vi "ScopeSignalManipulation_v1.vi"() -> ()   [LabVIEW 2018]
doc: "This example illustrates how to use autosetup and continuously acquires waveforms from a single channel using the following steps:\n\n1. Specify a valid VISA session. \n2. Specify a channel. \n3. Specify a time-out value for reading waveform.\n4. Run the VI. The graph displays the waveform you acquire."
uses:
  <vilib>/Analysis/baseanly.llb/Mean (DBL).vi
  <instrlib>/Tektronix DPO MSO 2000 4000 Series/Public/Data/Read (Single Waveform).vi
  <vilib>/Waveform/WDTFileIO.llb/Export Waveform To Spreadsheet File.vi
  <instrlib>/Tektronix DPO MSO 2000 4000 Series/Tektronix DPO MSO 2000 4000 Series.lvlib
  <vilib>/Analysis/NI_AALBase.lvlib
panel:
  in  "Tab Control":enum32{"Charge Amplifier", "Pulse Int"}(tab)=enum."Pulse Int"
  out "Charge Amp Signal (mV)":dbl=4.154735158126834 format="%#_6f"
  out "Number of Positrons":dbl=216046.22822259535
  out "Waveform Graph 2":waveform(dbl)(graph)={"t0"=timestamp(0 s since 1904-01-01), "dt"=4e-10, "Y"=array[5806 elements]}
  out "Base":dbl=-1.565120000000005e-08
  out "Signal":dbl=1.2079999999999996e-10
  out "Result (nVs)":dbl=15.77200000000005
  out "Mean BG":dbl=0.019374295870932312
  out "Mean ROI":dbl=0.015219560712805478
  out "BG ROI Length":i32=7314
  out "ROI Length":i32=2413
  out "I(BG Stop)":i32=495986
  out "I(BG start)":i32=488672
  out "I(stop)":i32=501340
  out "I(start)":i32=498927
  in  "Measurement Type":enum16{"Charge Amplifier", "Pulse Int"}(ring)=enum."Pulse Int"
  in  "Save waveform?":bool
  in  "acquire":bool=TRUE
  in  "milliseconds to wait":u32=100
  in  "Looping?":bool
  in  "stop":bool
  out "bkgd stop":dbl=0.000196584686774942
  out "bkgd start":dbl=0.00019546867749419954
  out "stop int":dbl=0.00020053596287703017
  out "start int":dbl=0.00019821345707656614
  in  "Channel (0: Channel 1)":u16(ring)=2 items=["Channel 1", "Channel 2", "Channel 3", "Channel 4", "Math", "Reference 1", "Reference 2", "Reference 3", "Reference 4"]
  in  "Maximum Time (10000ms)":u32=10000
  in  "VISA Resource Name":refnum<visa-resource-name>="mdo4034c"
  out "Waveform Graph":waveform(dbl)(graph)={"t0"=timestamp(-0.000197980000000042 s since 1904-01-01), "dt"=4e-10, "Y"=array[1000000 elements]}
  # "Region of Interest (ROI) Details"
  # "Time"
  # "Index"
  # "Length"
  # "Dashed cursors are the background, soild are the ROI"
  # "Use the solid ROI Cursors to define the region to integrate from the scope"
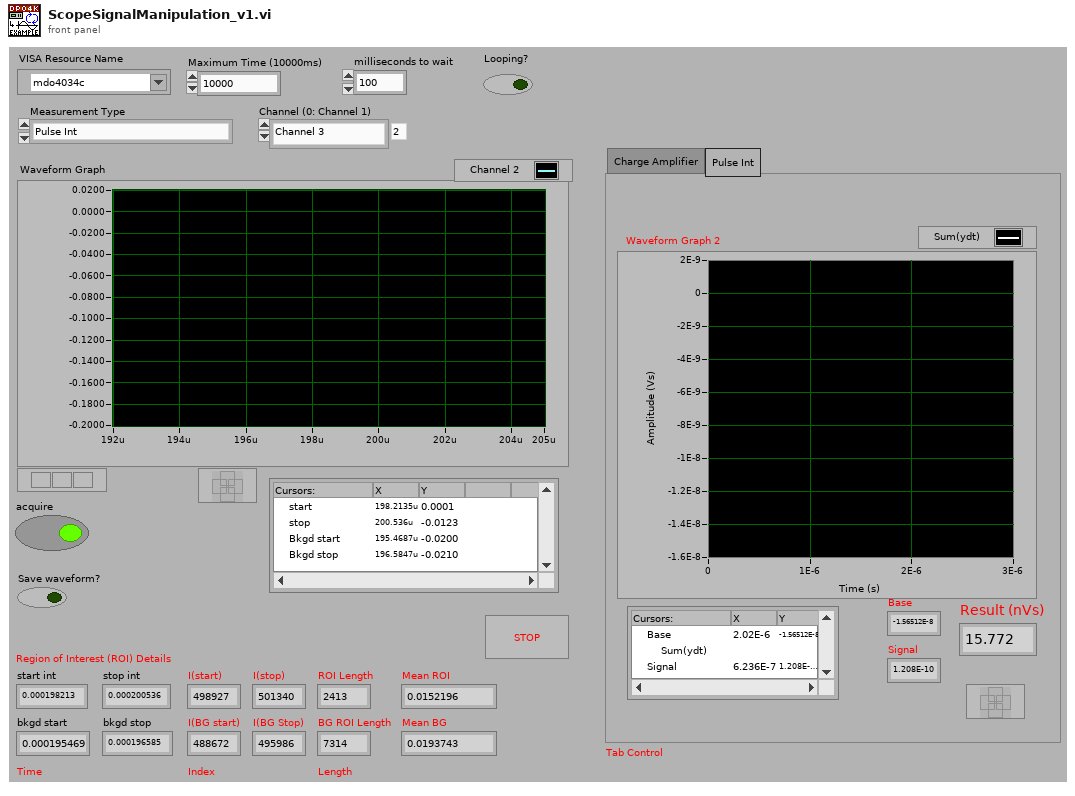
[diagram p1: front panel]
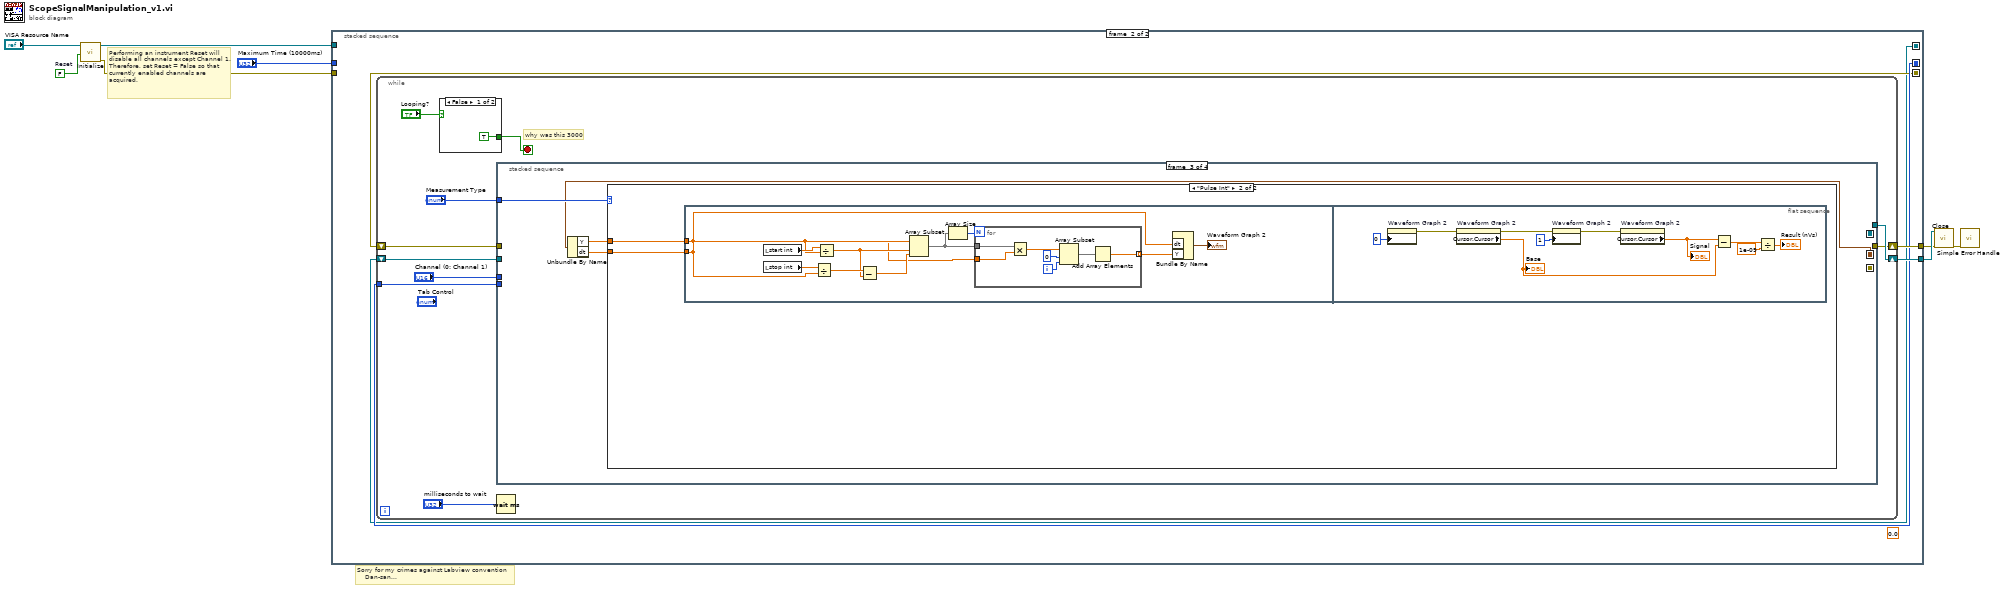
[diagram p0: block diagram]
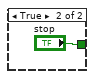
[diagram p3: hidden frame]
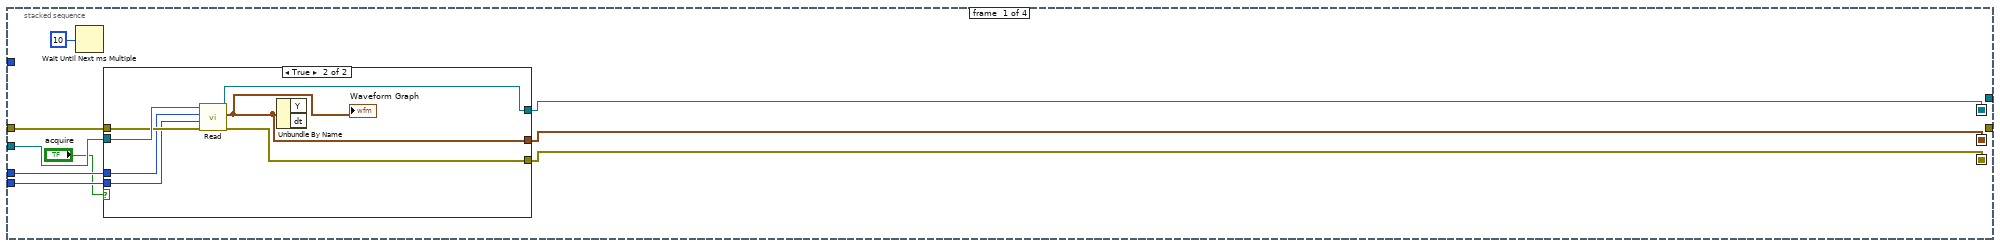
[diagram p4: hidden frame]
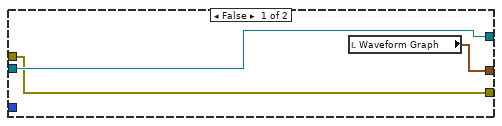
[diagram p5: hidden frame]
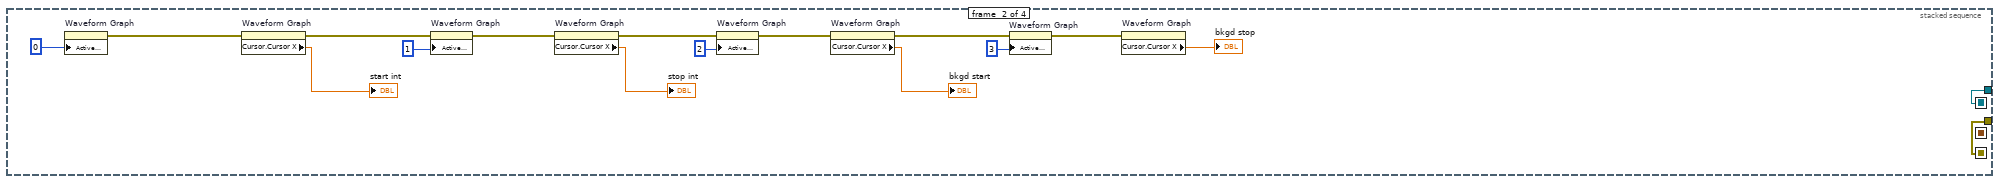
[diagram p6: hidden frame]
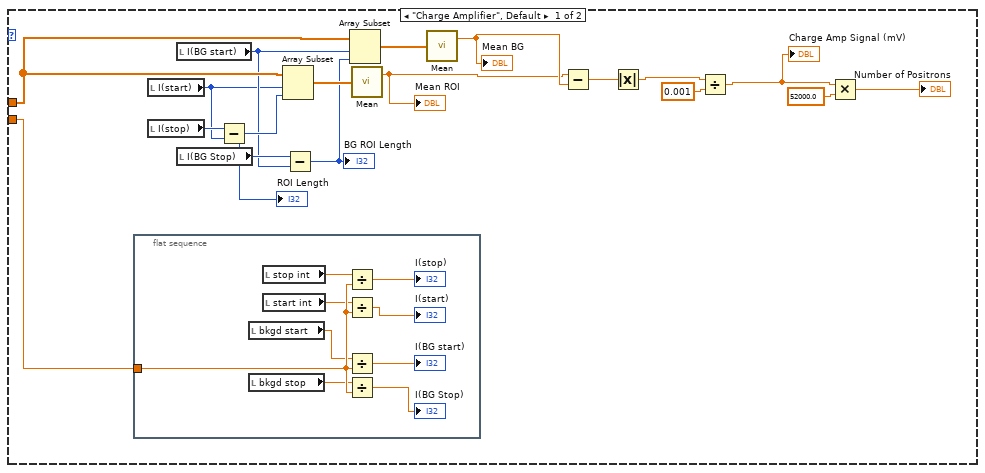
[diagram p7: hidden frame]
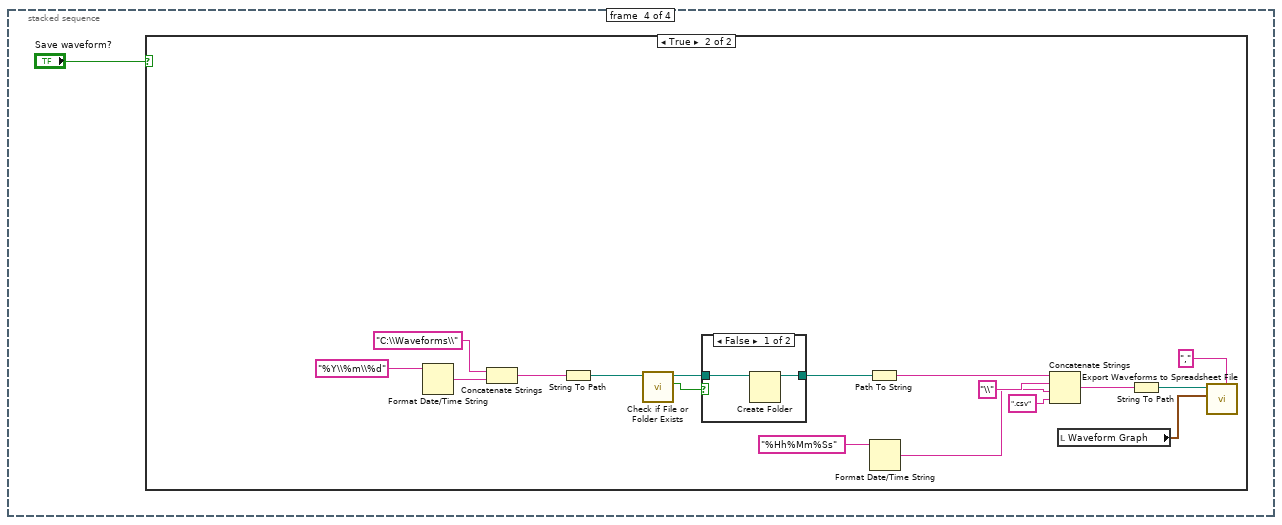
[diagram p8: hidden frame]
diagram:
  w4 = FALSE  # Reset
  # "Sorry for my crimes against Labview convention \n    Dan-san..."
  # "Performing an instrument Reset will disable all channels except Channel 1. Therefore, set Reset = False so that currently enabled channels are acquired."
  n1 = call <instrlib>:"Initialize.vi"("Reset (True)"=w4, "VISA resource name"="VISA Resource Name") -> ("error out"=w2:errorcluster, "VISA resource name out"=w1:refnum<visa-resource-name>)  [unwired: 8 in]
  n2 = stacked-sequence {
    seq-local: [w11 _] -> [_ w14]
    seq-local: [w10 _] -> [_ w13]
    seq-local: [w9 _] -> [_ w12]
    tunnel: "Maximum Time (10000ms)" -> [w11 _]
    tunnel: w2 -> [w10 _]
    tunnel: w1 -> [w9 _]
    tunnel: [_ w16] -> w7
    tunnel: [_ w15] -> w6
    frame #0 {
    }
    frame #1 {
      (unwired) 0.0
      n3 = while {
        tunnel: w14 -> [w24]
        shift-right: [w25] -> w15
        shift-left: w13 -> [w23]
        shift-right: [w26] -> w16
        shift-left: w12 -> [w22]
        stop <- w20 stop-if-true
        # "why was this 3000"
        n4 = case shown="False" "Looping?" {
          tunnel: [TRUE ("stop") "stop"] -> w20
          frame False {
          }
          frame True {
          }
        }
        n5 = stacked-sequence {
          seq-local: [w35 _ _ _] -> [_ w64 _ _]
          seq-local: [w33 _ _ _] -> [_ w63 _ _]
          seq-local: [w29 _ _ _] -> [_ _ w65 _]
          tunnel: w22 -> [w37 _ _ _]
          tunnel: w23 -> [w36 _ _ _]
          tunnel: w24 -> [w32 _ _ _]
          tunnel: "Channel (0: Channel 1)" -> [w31 _ _ _]
          tunnel: [_ w64 _ _] -> w26
          tunnel: [_ w63 _ _] -> w25
          tunnel: "Measurement Type" -> [_ _ w68 _]
          frame #0 {
            n6 = Wait Until Next ms Multiple(millisecond multiple=u32 10) -> ()  [unwired: 1 out]
            n7 = case shown="True" "acquire" {
              tunnel: w37 -> [w40 w47]
              tunnel: w36 -> [w39 w46]
              tunnel: [w40 w45] -> w35
              tunnel: [w39 w44] -> w33
              tunnel: w32 -> [_ w43]
              tunnel: w31 -> [_ w42]
              tunnel: [w38 w41] -> w29
              frame False {
                n8 = local read "Waveform Graph"() -> (w38:waveform(dbl))
              }
              frame True {
                n9 = call-poly <instrlib>:"Read.vi"("error in (no error)"=w46, "Maximum Time (10000ms)"=w43, "Channel (0: Channel 1)"=w42, "VISA resource name"=w47) -> ("error out"=w44:errorcluster, "Waveform Graph"=w41:waveform(dbl), "VISA resource name out"=w45:refnum<visa-resource-name>)  [unwired: 5 in]
                "Waveform Graph" <- w41
                n10 = Unbundle By Name(w41) -> ()  [unwired: 2 out]
              }
            }
          }
          frame #1 {
            n11 = property on="Waveform Graph" class="WFGraph (strict)"("Active Cursor"=0 ("Cursor.Cursor Index")) -> (error out=w61:errorcluster)  [unwired: 2 in, 1 out]
            n12 = property on="Waveform Graph" class="WFGraph (strict)"(error in=w61) -> (error out=w60:errorcluster, "Cursor.Cursor X"=→"start int":dbl)  [unwired: 1 in, 1 out]
            n13 = property on="Waveform Graph" class="WFGraph (strict)"(error in=w60, "Active Cursor"=1 ("Cursor.Cursor Index")) -> (error out=w59:errorcluster)  [unwired: 1 in, 1 out]
            n14 = property on="Waveform Graph" class="WFGraph (strict)"(error in=w59) -> (error out=w54:errorcluster, "Cursor.Cursor X"=→"stop int":dbl)  [unwired: 1 in, 1 out]
            n15 = property on="Waveform Graph" class="WFGraph (strict)"(error in=w54, "Active Cursor"=u32 2) -> (error out=w55:errorcluster)  [unwired: 1 in, 1 out]
            n16 = property on="Waveform Graph" class="WFGraph (strict)"(error in=w55) -> (error out=w51:errorcluster, "Cursor.Cursor X"=→"bkgd start":dbl)  [unwired: 1 in, 1 out]
            n17 = property on="Waveform Graph" class="WFGraph (strict)"(error in=w51, "Active Cursor"=u32 3) -> (error out=w52:errorcluster)  [unwired: 1 in, 1 out]
            n18 = property on="Waveform Graph" class="WFGraph (strict)"(error in=w52) -> ("Cursor.Cursor X"=→"bkgd stop":dbl)  [unwired: 1 in, 2 out]
          }
          frame #2 {
            n19 = Unbundle By Name(w65) -> ("Y"=w66:dbl[], "dt"=w67:dbl)
            n20 = case shown="\"Pulse Int\"" w68 {
              tunnel: w67 -> [w86 w96]
              tunnel: w66 -> [w83 w97]
              frame "Charge Amplifier", Default {
                n21 = flat-sequence {
                  tunnel: w86 -> [w95]
                  frame #0 {
                    n22 = local read "bkgd start"() -> (w92:dbl)
                    n23 = local read "bkgd stop"() -> (w93:dbl)
                    n24 = local read "stop int"() -> (w94:dbl)
                    n25 = local read "start int"() -> (w91:dbl)
                    n26 = Divide(x=w94, y=w95) -> (x/y=→"I(stop)":dbl)
                    n27 = Divide(x=w91, y=w95) -> (x/y=→"I(start)":dbl)
                    n28 = Divide(x=w92, y=w95) -> (x/y=→"I(BG start)":dbl)
                    n29 = Divide(x=w93, y=w95) -> (x/y=→"I(BG Stop)":dbl)
                  }
                }
                n30 = local read "I(start)"() -> (w76:i32)
                n31 = local read "I(stop)"() -> (w79:i32)
                n32 = local read "I(BG start)"() -> (w77:i32)
                n33 = local read "I(BG Stop)"() -> (w78:i32)
                n34 = Subtract(x=w79, y=w76) -> (x-y=w85:i32)
                "ROI Length" <- w85
                n35 = Array Subset(array=w83, index=w76, length=w85) -> (w84:dbl[])
                n36 = Subtract(x=w78, y=w77) -> (x-y=w69:i32)
                "BG ROI Length" <- w69
                n37 = Array Subset(array=w83, index=w77, length=w69) -> (w82:dbl[])
                n38 = call-poly <vilib>:"Mean.vi"("X"=w84) -> ("mean"=w80:dbl)  [unwired: 1 out]
                "Mean ROI" <- w80
                n39 = call-poly <vilib>:"Mean.vi"("X"=w82) -> ("mean"=w81:dbl)  [unwired: 1 out]
                "Mean BG" <- w81
                n40 = Subtract(x=w80, y=w81) -> (x-y=w73:dbl)
                n41 = Absolute Value(x=w73) -> (abs(x)=w72:dbl)
                n42 = Divide(x=w72, y=0.001) -> (x/y=w70:dbl)
                "Charge Amp Signal (mV)" <- w70
                n43 = Multiply(x=w70, y=52000.0) -> (x*y=→"Number of Positrons":dbl)
              }
              frame "Pulse Int" {
                n44 = flat-sequence {
                  tunnel: w97 -> [w105]
                  tunnel: w96 -> [w98]
                  frame #0 {
                    n45 = local read "start int"() -> (w103:dbl)
                    n46 = local read "stop int"() -> (w104:dbl)
                    n47 = Divide(x=w104, y=w98) -> (x/y=w102:dbl)
                    n48 = Divide(x=w103, y=w98) -> (x/y=w101:dbl)
                    n49 = Subtract(x=w102, y=w101) -> (x-y=w100:dbl)
                    n50 = Array Subset(array=w105, index=w101, length=w100) -> (w99:dbl[])
                    n51 = Array Size(array=w99) -> (size(s)=w108:i32)
                    n52 = for {
                      N: w108 -> [_]
                      tunnel: w99 -> [w111]
                      tunnel: [w112] -> w107 mode=indexing
                      tunnel: w98 -> [w110]
                      i -> [w114]
                      n53 = Multiply(x=w111, y=w110) -> (x*y=w109:dbl[])
                      n54 = Array Subset(array=w109, index=0, length=w114) -> (w113:dbl[])
                      n55 = Add Array Elements(numeric array=w113) -> (sum=w112:dbl)
                    }
                    n56 = Bundle By Name("dt"=w98, "Y"=w107) -> (→"Waveform Graph 2":waveform(dbl))  [unwired: 1 in]
                  }
                  frame #1 {
                    n57 = property on="Waveform Graph 2" class="WFGraph (strict)"("Active Cursor"=u32 0) -> (error out=w124:errorcluster)  [unwired: 2 in, 1 out]
                    n58 = property on="Waveform Graph 2" class="WFGraph (strict)"(error in=w124) -> (error out=w121:errorcluster, "Cursor.Cursor Y"=w119:dbl)  [unwired: 1 in, 1 out]
                    "Base" <- w119
                    n59 = property on="Waveform Graph 2" class="WFGraph (strict)"(error in=w121, "Active Cursor"=u32 1) -> (error out=w122:errorcluster)  [unwired: 1 in, 1 out]
                    n60 = property on="Waveform Graph 2" class="WFGraph (strict)"(error in=w122) -> ("Cursor.Cursor Y"=w120:dbl)  [unwired: 1 in, 2 out]
                    "Signal" <- w120
                    n61 = Subtract(x=w120, y=w119) -> (x-y=w118:dbl)
                    n62 = Divide(x=w118, y=1e-09) -> (x/y=→"Result (nVs)":dbl)
                  }
                }
              }
            }
          }
          frame #3 {
            n63 = case shown="True" "Save waveform?" {
              frame False {
              }
              frame True {
                n64 = Format Date/Time String(time format string (%c)="%Y\\%m\\%d") -> (date/time string=w140:string)  [unwired: 2 in]
                n65 = Concatenate Strings("C:\\Waveforms\\" ("string"), w140) -> (w141:string)
                n66 = String To Path(string=w141) -> (path=w138:path)
                n67 = call <vilib>:"Check if File or Folder Exists.vi"("path"=w138) -> ("file or folder exists?"=w136:bool, "dup path"=w135:path)  [unwired: 8 in, 1 out]
                n68 = case shown="False" w136 {
                  tunnel: w135 -> [w145 w146]
                  tunnel: [w144 w146] -> w134
                  frame False {
                    n69 = Create Folder(path (use dialog)=w145) -> (created path=w144:path)  [unwired: 2 in, 2 out]
                  }
                  frame True {
                  }
                }
                n70 = Path To String(path=w134) -> (string=w133:string)
                n71 = Format Date/Time String(time format string (%c)="%Hh%Mm%Ss") -> (date/time string=w130:string)  [unwired: 2 in]
                n72 = Concatenate Strings(w133, "\\" ("string"), w130, ".csv" ("string")) -> (w129:string)
                n73 = local read "Waveform Graph"() -> (w143:waveform(dbl))
                n74 = String To Path(string=w129) -> (path=w128:path)
                n75 = call-poly <vilib>:"Export Waveforms to Spreadsheet File.vi"("delimiter (Tab)"=",", "waveform"=w143, "file path (dialog if empty)"=w128) -> ()  [unwired: 7 in, 2 out]
              }
            }
          }
        }
        n76 = Wait (ms)(milliseconds to wait="milliseconds to wait") -> ()  [unwired: 1 out]
      }
    }
  }
  n77 = call <instrlib>:"Close.vi"("error in (no error)"=w6, "VISA resource name"=w7) -> ("error out"=w5:errorcluster)  [unwired: 9 in]
  n78 = call <vilib>:"Simple Error Handler.vi"("error in (no error)"=w5) -> ()  [unwired: 4 in, 5 out]
